vi "Write Init each cycle.vi"(8 "error in (no error)":errorcluster, 10 "Init each cycle":bool=TRUE, 11 "Keithley 622x2182 Driver in":refnum<class "Keithley 622x2182 Driver.lvclass">) -> (0 "error out":errorcluster, 3 "Keithley 622x2182 Driver out":refnum<class "Keithley 622x2182 Driver.lvclass">)   [LabVIEW 2021, in "Keithley 622x2182 Driver.lvclass"]
uses:
  Keithley 622x2182 Driver.lvclass
  Keithley 622x2182 Driver.lvclass/Keithley 622x2182 Driver.ctl
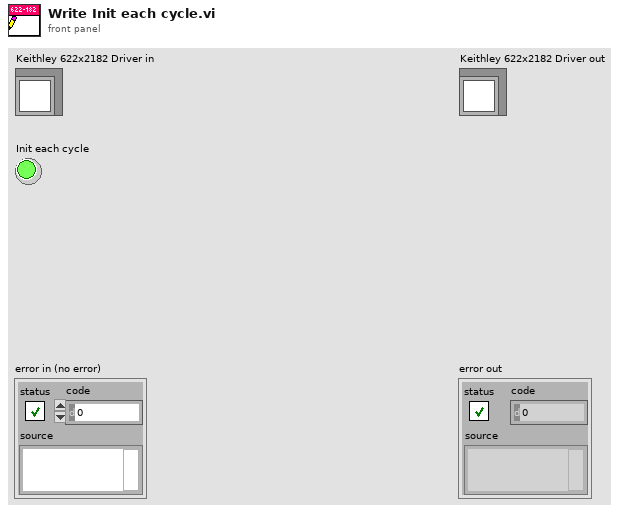
[diagram p1: front panel]
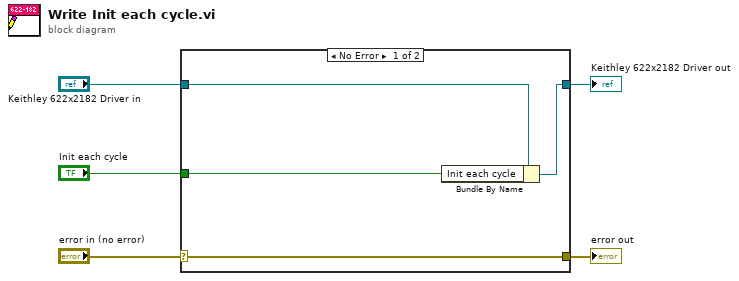
[diagram p0: block diagram]
diagram:
  n1 = case shown="No Error" "error in (no error)" {
    selector: "error in (no error)" -> [w9 w10]
    tunnel: [w9 w10] -> w4
    tunnel: [w7 w11] -> w2
    tunnel: "Keithley 622x2182 Driver in" -> [w8 w11]
    tunnel: "Init each cycle" -> [w6 _]
    frame No Error {
      n2 = Bundle By Name(cluster=w8, "Init each cycle"=w6) -> (w7:refnum<class "Keithley 622x2182 Driver.lvclass">)
    }
    frame Error {
    }
  }
  "error out" <- w4
  "Keithley 622x2182 Driver out" <- w2
